vi "Vsolver_destructor.vi"(8 "error in (no error)":errorcluster, 11 "Vsolver in":refnum<class "Vsolver.lvclass">) -> (0 "error out":errorcluster, 3 "Vsolver out":refnum<class "Vsolver.lvclass">)   [LabVIEW 2020, in "Sgraph_lib_V1.lvlib" / "Vsolver.lvclass"]
doc: "Close reference to Vsolver class"
uses:
  Vsolver.lvclass
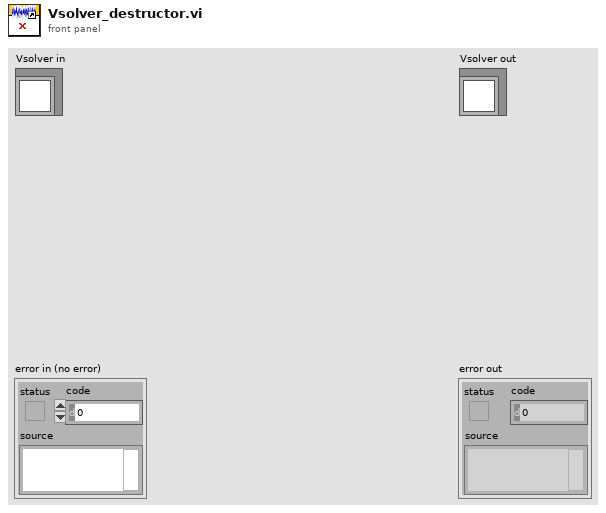
[diagram p1: front panel]
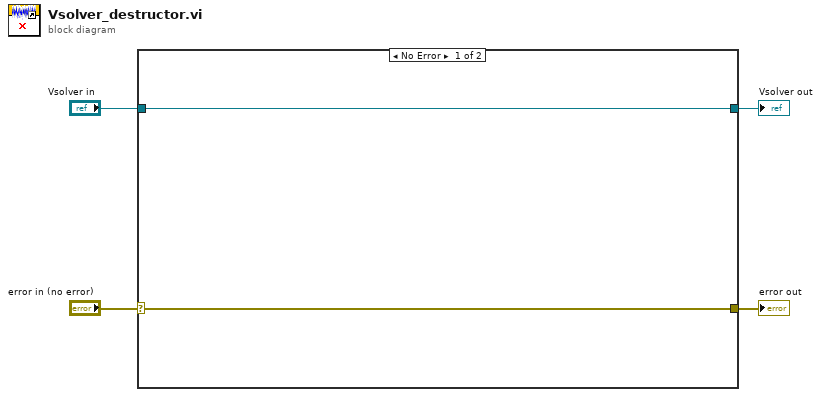
[diagram p0: block diagram]
diagram:
  n1 = case shown="No Error" "error in (no error)" {
    selector: "error in (no error)" -> [w5 w8]
    tunnel: [w5 w8] -> w3
    tunnel: [w6 w7] -> w1
    tunnel: "Vsolver in" -> [w6 w7]
    frame No Error {
    }
    frame Error {
    }
  }
  "error out" <- w3
  "Vsolver out" <- w1
